vi "Add Metadata.vi"(6 "Location":string, 8 "error in (no error)":errorcluster, 9 "Reset":bool, 10 "Metadata":refnum<class "Metadata.lvclass">[](array[class]), 11 "Worker in":refnum<class "Worker Actor.lvclass">) -> (0 "error out":errorcluster, 3 "Worker out":refnum<class "Worker Actor.lvclass">)   [LabVIEW 2021, in "Worker Actor.lvclass"]
uses:
  Worker Actor.lvclass
  NHMFL_Core/Libraries/File/Metadata/Metadata.lvclass
  Worker Actor.lvclass/Worker Actor.ctl
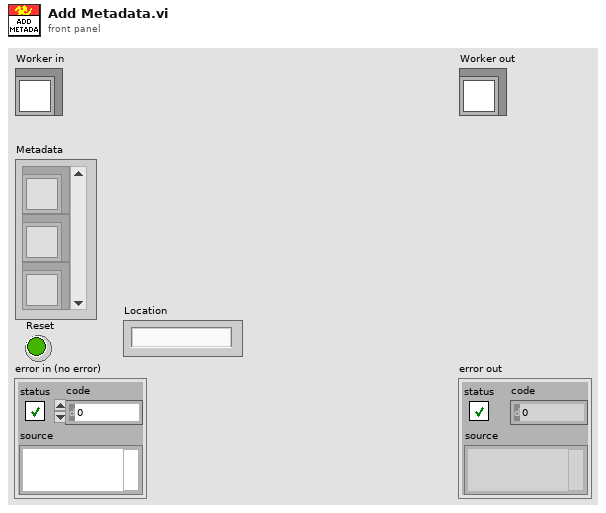
[diagram p1: front panel]
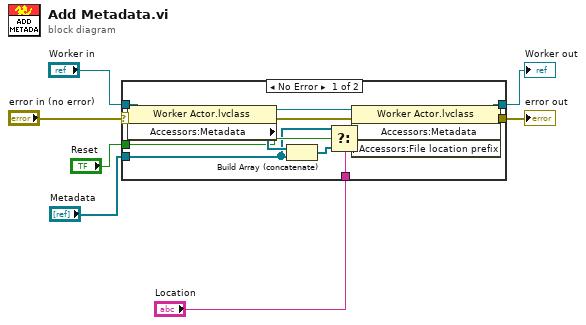
[diagram p0: block diagram]
diagram:
  n1 = case shown="No Error" "error in (no error)" {
    selector: "error in (no error)" -> [w19 w21]
    tunnel: [w16 w21] -> w6
    tunnel: [w14 w20] -> w4
    tunnel: "Worker in" -> [w17 w20]
    tunnel: "Metadata" -> [w11 _]
    tunnel: "Reset" -> [w12 _]
    tunnel: "Location" -> [w8 _]
    frame No Error {
      n2 = property class="Worker Actor.lvclass"(reference=w17, error in=w19) -> (reference out=w15:refnum<class "Worker Actor.lvclass">, error out=w18:errorcluster, "Accessors:Metadata"=w13:refnum<class "Metadata.lvclass">[])
      n3 = Build Array (concatenate)(w13, w11) -> (w10:refnum<class "Metadata.lvclass">[])
      n4 = Select(t=w11, s=w12, f=w10) -> (s? t:f=w9:refnum<class "Metadata.lvclass">[])
      n5 = property class="Worker Actor.lvclass"(reference=w15, error in=w18, "Accessors:Metadata"=w9, "Accessors:File location prefix"=w8) -> (reference out=w14:refnum<class "Worker Actor.lvclass">, error out=w16:errorcluster)
    }
    frame Error {
    }
  }
  "error out" <- w6
  "Worker out" <- w4
